vi "EquiRipple Filter Design.vi"() -> ()   [LabVIEW 2017]
doc: "This example shows the Transfer Function of an EquiRipple FIR filter given the Filter Type chosen by the user. \n\nThe parameters are different for each type and may be changed to investigate their effect on the response."
uses:
  <vilib>/Utility/error.llb/DialogType.ctl
  <vilib>/Analysis/3filter.llb/Equi-Ripple LowPass (DBL).vi
  <vilib>/Analysis/3filter.llb/Equi-Ripple HighPass (DBL).vi
  <vilib>/Analysis/3filter.llb/Equi-Ripple BandPass (DBL).vi
  <vilib>/Analysis/3filter.llb/Equi-Ripple BandStop (DBL).vi
  <vilib>/measure/NI_MAPro.lvlib
  <vilib>/Analysis/NI_AALBase.lvlib
  <vilib>/Analysis/NI_AALPro.lvlib
panel:
  out "Error Message":string
  in  "Stop":bool
  in  "Filter Type":T1(tab)
  in  "pass frequency":dbl=200.0
  in  "stop frequency":dbl=300.0
  in  "pass frequency":dbl=300.0 format="%#.6g"
  in  "stop frequency":dbl=200.0 format="%#.6g"
  in  "low pass frequency":dbl=200.0 format="%#.6g"
  in  "high pass frequency":dbl=300.0 format="%#.6g"
  in  "low stop frequency":dbl=100.0 format="%#.6g"
  in  "high stop frequency":dbl=400.0 format="%#.6g"
  in  "high stop frequency":dbl=300.0 format="%#.6g"
  in  "low stop frequency":dbl=200.0 format="%#.6g"
  in  "high pass frequency":dbl=400.0 format="%#.6g"
  in  "low pass frequency":dbl=100.0 format="%#.6g"
  out "Phase Response":cluster{dbl, dbl, dbl[]}(graph)
  out "Magnitude Response":cluster{dbl, dbl, dbl[]}(graph)
  in  "sampling rate":dbl=1000.0 format="%#.6g"
  in  "No. of Taps":i32=30
  # "Overview: Demonstrates the specification of lowpass, highpass, bandpass, and bandstop filters.\nRequirements: LabVIEW Full Development System\nInstructions: \n1. Run the VI.\n2. Interact with the filter settings, noting any error messages that occur for invalid settings.\n3. Click Stop to stop the VI."
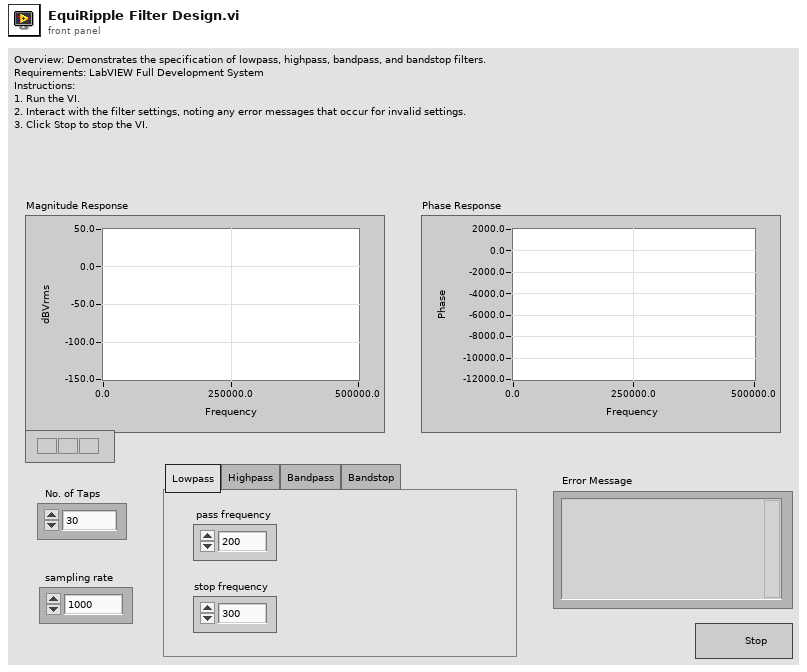
[diagram p1: front panel]
types:
  T1 = enum32{"Lowpass", "Highpass", "Bandpass", "Bandstop"}
  T2 = enum32{"Vrms", "Vpk", "Vrms^2", "Vpk^2", "Vrms/rtHz", "Vpk/rtHz", "Vrms^2/Hz", "Vpk^2/Hz"}
  T3 = enum16{"Power (Vrms^2)", "Amplitude (Vrms)", "Gain (amplitude ratio)"}
  T4 = typedef "DialogType.ctl" = u16
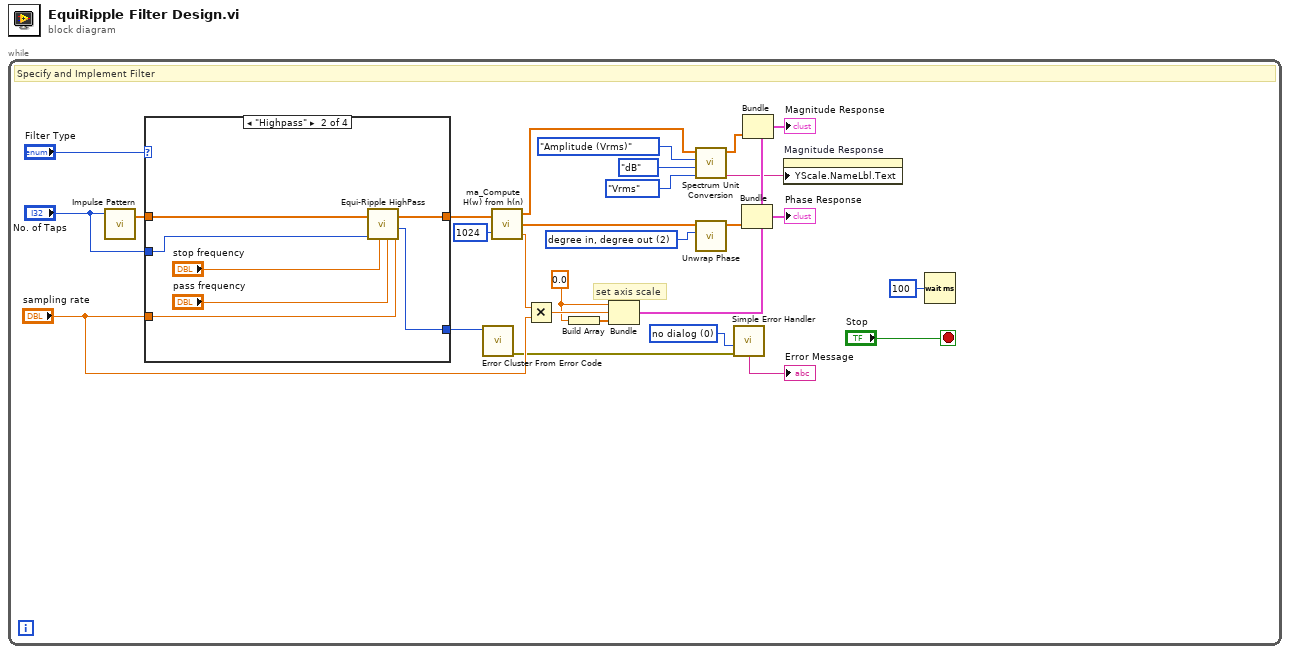
[diagram p0: block diagram]
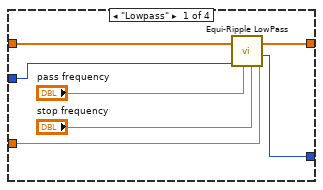
[diagram p2: hidden frame]
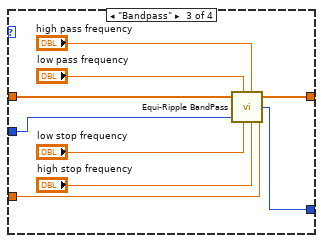
[diagram p3: hidden frame]
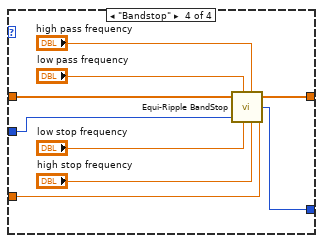
[diagram p4: hidden frame]
diagram:
  n1 = while {
    stop <- "Stop" stop-if-true
    w2 = 0.0
    w5 = 2 items=["radian in, radian out", "radian in, degree out", "degree in, degree out", "degree in, radian out"] ("phase unit")
    w10 = T4 0 items=["no dialog", "OK message", "continue or stop message", "OK message + warnings", "continue/stop + warnings"] ("type of dialog (OK msg:1)")
    # "set axis scale"
    # "Specify and Implement Filter"
    n2 = call <vilib>:"Impulse Pattern.vi"("samples"="No. of Taps") -> ("Impulse Pattern"=w17:dbl[])  [unwired: 2 in, 1 out]
    n3 = case shown="\"Highpass\"" "Filter Type" {
      tunnel: "No. of Taps" -> [w33 w40 w49 w52]
      tunnel: w17 -> [w34 w41 w50 w59]
      tunnel: [w35 w42 w51 w60] -> w8
      tunnel: "sampling rate" -> [w32 w39 w48 w58]
      tunnel: [w31 w36 w43 w53] -> w13
      frame "Lowpass" {
        n4 = call-poly <vilib>:"Equi-Ripple LowPass.vi"("# of taps"=w33, "pass freq"="pass frequency", "stop freq"="stop frequency", "sampling freq: fs"=w32, "X"=w34) -> ("error"=w31:i32, "Filtered X"=w35:dbl[])  [unwired: 1 in]
      }
      frame "Highpass" {
        n5 = call-poly <vilib>:"Equi-Ripple HighPass.vi"("# of taps"=w40, "stop freq"="stop frequency", "high freq"="pass frequency", "sampling freq: fs"=w39, "X"=w41) -> ("error"=w36:i32, "Filtered X"=w42:dbl[])  [unwired: 1 in]
      }
      frame "Bandpass" {
        n6 = call-poly <vilib>:"Equi-Ripple BandPass.vi"("X"=w50, "lower pass freq"="low pass frequency", "# of taps"=w49, "lower stop freq"="low stop frequency", "higher pass freq"="high pass frequency", "higher stop freq"="high stop frequency", "sampling freq: fs"=w48) -> ("Filtered X"=w51:dbl[], "error"=w43:i32)  [unwired: 1 in]
      }
      frame "Bandstop" {
        n7 = call-poly <vilib>:"Equi-Ripple BandStop.vi"("X"=w59, "lower pass freq"="low pass frequency", "# of taps"=w52, "lower stop freq"="low stop frequency", "higher pass freq"="high pass frequency", "higher stop freq"="high stop frequency", "sampling freq: fs"=w58) -> ("Filtered X"=w60:dbl[], "error"=w53:i32)  [unwired: 1 in]
      }
    }
    n8 = call <vilib>:"Error Cluster From Error Code.vi"("error code (0)"=w13) -> ("error out"=w11:errorcluster)  [unwired: 8 in]
    n9 = call <vilib>:"ma_Compute H(w) from h(n).vi"("h"=w8, "FFT size"=1024) -> ("Mag H(w)"=w7:dbl[], "Phase H(w)"=w6:dbl[], "df"=w24:dbl)
    n10 = Multiply(x=w24, y="sampling rate") -> (x*y=w23:dbl)
    n11 = Build Array ("array")(w2) -> (w28:dbl[])
    n12 = Bundle(w2, w23, w28) -> (w26:cluster{dbl, dbl, dbl[]})  [unwired: 1 in]
    n13 = call <vilib>:"Spectrum Unit Conversion.vi"("display unit"=T2."Vrms", "log/linear"=enum16{"Linear", "dB", "dBm"}."dB", "spectrum type"=T3."Amplitude (Vrms)", "Spectrum in"=w7) -> ("spectrum unit"=w18:string, "Spectrum out"=w21:dbl[])  [unwired: 6 in]
    n14 = call <vilib>:"Unwrap Phase.vi"("phase unit"=w5, "Phase"=w6) -> ("Unwrapped Phase"=w4:dbl[])  [unwired: 8 in, 1 out]
    n15 = call <vilib>:"Simple Error Handler.vi"("type of dialog (OK msg:1)"=w10, "error in (no error)"=w11) -> ("message"=→"Error Message":string)  [unwired: 3 in, 4 out]
    n16 = Bundle(cluster=w26, w4) -> (→"Phase Response":cluster{dbl, dbl, dbl[]})  [unwired: 2 in]
    n17 = Bundle(cluster=w26, w21) -> (→"Magnitude Response":cluster{dbl, dbl, dbl[]})  [unwired: 2 in]
    n18 = property on="Magnitude Response" class="WFGraph (엄격한)"("YScale.NameLbl.Text"=w18) -> ()  [unwired: 2 in, 2 out]
    n19 = Wait (ms)(milliseconds to wait=u32 100) -> ()  [unwired: 1 out]
  }
